vi "Configure Limit Line.vi"(0 "VISA resource name":refnum<visa-resource-name>, 1 "Enable Limit (T: Enable)":bool=TRUE, 2 "Enable Test (T: Enable)":bool=TRUE, 3 "Limit Type (0: Upper)":u16(ring) items=["Upper", "Lower"], 5 "Limit Line (1: Line1)":u16(ring)=1 items=["Line1"=1, "Line2"=2], 7 "Enable Margin (T: Enable)":bool=TRUE, 9 "Manual Margin (0 dB)":dbl, 11 "error in (no error)":errorcluster, 12 "Amplitude Interpolation (0: Linear)":u16(ring) items=["Linear", "Logarithmic"], 13 "Frequency Interpolation (0: Linear)":u16(ring) items=["Linear", "Logarithmic"]) -> (4 "VISA resource name out":refnum<visa-resource-name>, 15 "error out":errorcluster)   [LabVIEW 2014, in "Agilent ESA PSA Series.lvlib"]
doc: "Configures limit line and allows you to enable limit line testing."
uses:
  Agilent ESA PSA Series.lvlib
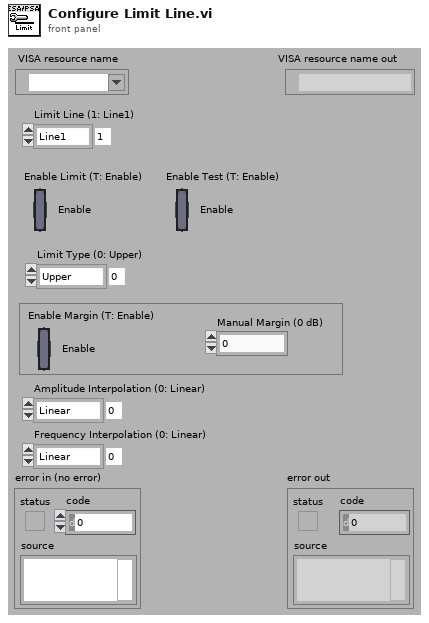
[diagram p1: front panel]
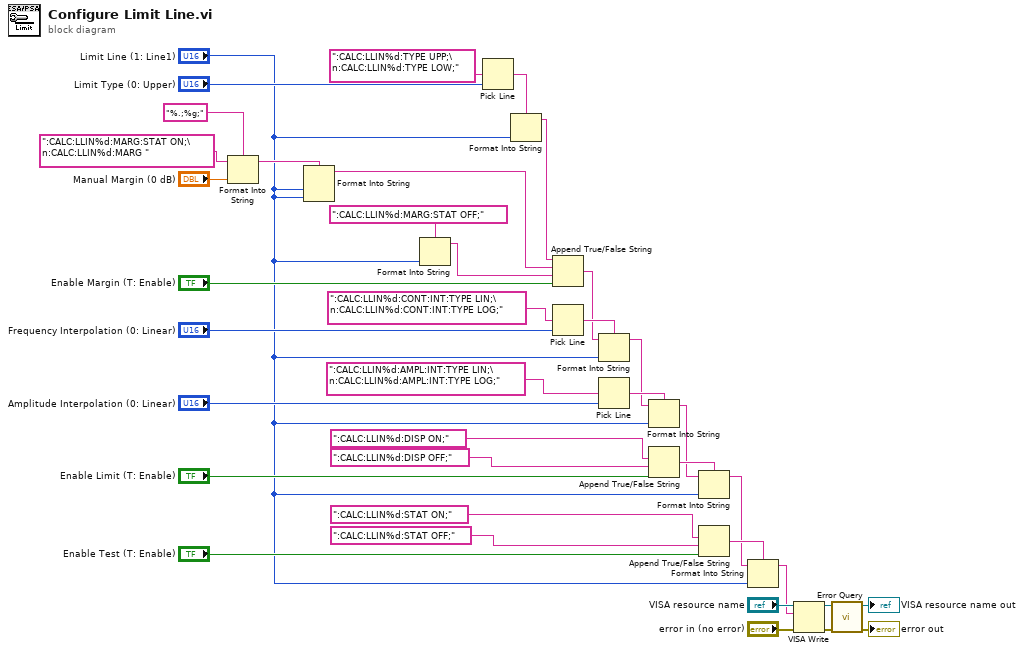
[diagram p0: block diagram]
diagram:
  n1 = Format Into String(format string="%.;%g;", initial string=":CALC:LLIN%d:MARG:STAT ON;\n:CALC:LLIN%d:MARG " ("format string"), "Manual Margin (0 dB)") -> (resulting string=w3:string)  [unwired: 1 in, 1 out]
  n2 = Format Into String(format string=w3, "Limit Line (1: Line1)", "Limit Line (1: Line1)") -> (resulting string=w6:string)  [unwired: 2 in, 1 out]
  n3 = Format Into String(format string=":CALC:LLIN%d:MARG:STAT OFF;", "Limit Line (1: Line1)") -> (resulting string=w7:string)  [unwired: 2 in, 1 out]
  n4 = Pick Line(multi-line string=":CALC:LLIN%d:TYPE UPP;\n:CALC:LLIN%d:TYPE LOW;", line index="Limit Type (0: Upper)") -> (output string=w5:string)  [unwired: 1 in]
  n5 = Format Into String(format string=w5, "Limit Line (1: Line1)") -> (resulting string=w2:string)  [unwired: 2 in, 1 out]
  n6 = Append True/False String(1:"Enable Margin (T: Enable)", 2:w7, 3:w6, 4:w2) -> (0:w4:string)
  n7 = Pick Line(multi-line string=":CALC:LLIN%d:CONT:INT:TYPE LIN;\n:CALC:LLIN%d:CONT:INT:TYPE LOG;", line index="Frequency Interpolation (0: Linear)") -> (output string=w23:string)  [unwired: 1 in]
  n8 = Format Into String(format string=w23, initial string=w4, "Limit Line (1: Line1)") -> (resulting string=w19:string)  [unwired: 1 in, 1 out]
  n9 = Pick Line(multi-line string=":CALC:LLIN%d:AMPL:INT:TYPE LIN;\n:CALC:LLIN%d:AMPL:INT:TYPE LOG;", line index="Amplitude Interpolation (0: Linear)") -> (output string=w20:string)  [unwired: 1 in]
  n10 = Format Into String(format string=w20, initial string=w19, "Limit Line (1: Line1)") -> (resulting string=w14:string)  [unwired: 1 in, 1 out]
  n11 = Append True/False String(1:"Enable Limit (T: Enable)", 2:":CALC:LLIN%d:DISP OFF;" ("false string"), 3:":CALC:LLIN%d:DISP ON;" ("false string")) -> (0:w15:string)  [unwired: 1 in]
  n12 = Format Into String(format string=w15, initial string=w14, "Limit Line (1: Line1)") -> (resulting string=w9:string)  [unwired: 1 in, 1 out]
  n13 = Append True/False String(1:"Enable Test (T: Enable)", 2:":CALC:LLIN%d:STAT OFF;" ("true string"), 3:":CALC:LLIN%d:STAT ON;" ("true string")) -> (0:w10:string)  [unwired: 1 in]
  n14 = Format Into String(format string=w10, initial string=w9, "Limit Line (1: Line1)") -> (resulting string=w8:string)  [unwired: 1 in, 1 out]
  n15 = VISA Write(VISA resource name="VISA resource name", write buffer=w8, error in (no error)="error in (no error)") -> (VISA resource name out=w36:refnum<visa-resource-name>, error out=w34:errorcluster)  [unwired: 1 out]
  n16 = call "Error Query.vi"("error in (no error)"=w34, "VISA resource name"=w36) -> ("error out"=→"error out":errorcluster, "VISA resource name out"=→"VISA resource name out":refnum<visa-resource-name>)  [unwired: 6 in, 2 out]
